vi "Low-Level HTTP Request AWS v4.vi"(5 "AWS Core":refnum<class "HTTP Request.lvclass">, 7 "Request Options":T2, 8 "error in (no error)":errorcluster, 9 "URL Suffix":string, 10 "URL Prefix":string, 11 "HTTP-Verb":string(combo)="GET") -> (0 "error out":errorcluster, 2 "Response":T1, 3 "Call Result":string)   [LabVIEW 2015, in "NI_AWS_Core.lvlib" / "HTTP Request.lvclass"]
doc: "This core implementation of AWS v4 HTTP requests may be used to implement special requests or API calls not present in this toolkit."
uses:
  HTTP Request.lvclass
  Request Options.ctl
  Name Value Pair.ctl
  Response.ctl
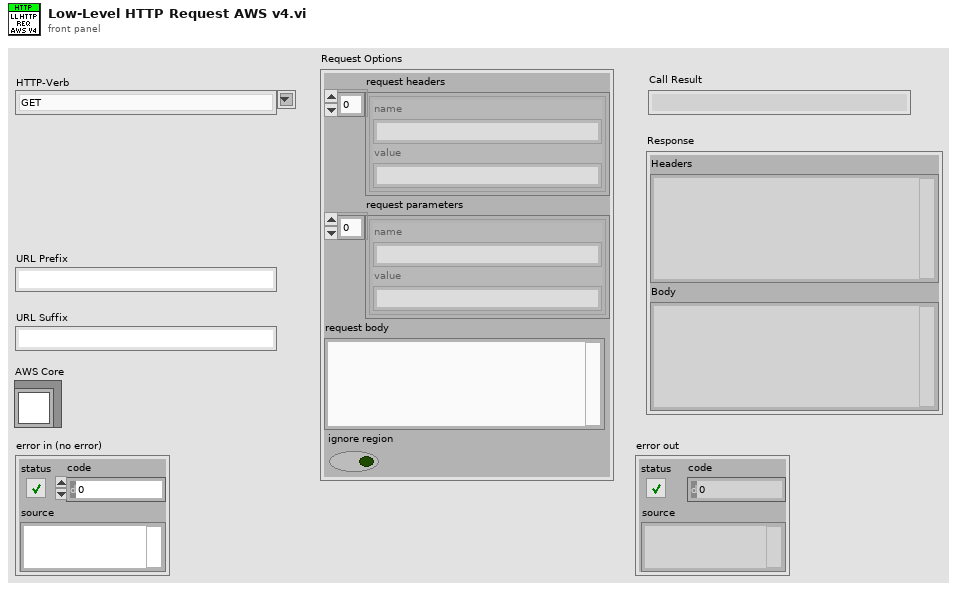
[diagram p1: front panel]
types:
  T1 = typedef "NI_AWS_Core.lvlib/HTTP Request.lvclass/Response.ctl" = cluster{"Headers":string, "Body":string}
  T2 = typedef "NI_AWS_Core.lvlib/HTTP Request.lvclass/Request Options.ctl" = cluster{"request headers":T3[], "request parameters":T3[], "request body":string, "ignore region":bool}
  T3 = typedef "NI_AWS_Core.lvlib/HTTP Request.lvclass/Name Value Pair.ctl" = cluster{"name":string, "value":string}
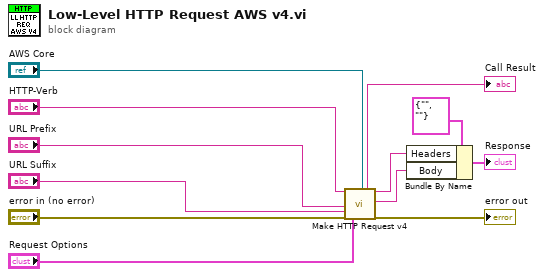
[diagram p0: block diagram]
diagram:
  n1 = call "Make HTTP Request v4.vi"("HTTP-Verb"="HTTP-Verb", "URL Prefix"="URL Prefix", "URL Suffix"="URL Suffix", "error in"="error in (no error)", "Request Options"="Request Options", "AWS Core"="AWS Core") -> ("Call Result"=→"Call Result":string, "response headers"=w5:string, "response body"=w4:string, "error out"=→"error out":errorcluster)  [unwired: 10 in]
  n2 = Bundle By Name(cluster=T1 {"Headers"="", "Body"=""} ("Response"), "Headers"=w5, "Body"=w4) -> (→"Response":T1)
